vi "Create Type.vi"(6 "Searchable Attributes":string[](array[string]), 8 "error in (no error)":errorcluster, 9 "Description":string, 10 "Name":string, 11 "IoT Session in":refnum<class "IoT Session.lvclass">) -> (0 "error out":errorcluster, 3 "IoT Session out":refnum<class "IoT Session.lvclass">)   [LabVIEW 2015, in "NI_AWS_IoT.lvlib" / "IoT Session.lvclass"]
uses:
  IoT Session.lvclass
  Core/HTTP Request/Valid String Specification.ctl
  Core/HTTP Request/Request Options.ctl
  Core/HTTP Request/Name Value Pair.ctl
  Core/HTTP Request/Region handling.ctl
  Core/HTTP Request/URL formatting.ctl
  Core/HTTP Request/HTTP Request.lvclass
  JSON Parsing/NI_JSON Parsing.lvlib
panel:
  out "Created Type ARN":string
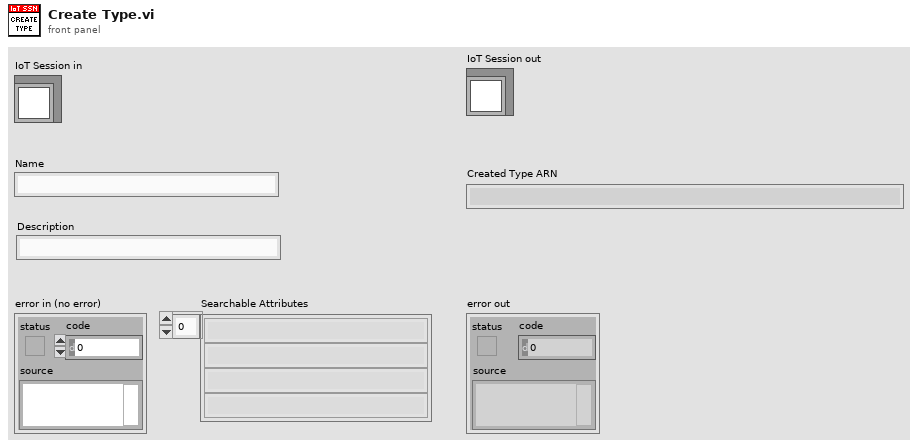
[diagram p1: front panel]
types:
  T1 = typedef "NI_AWS_Core.lvlib/HTTP Request.lvclass/Valid String Specification.ctl" = enum16{"none", "only [alphanumeric][-][_]", "only [alphanumeric][-][_][space]", "phone number +1xxxyyyzzzz", "Regular Expression"}
  T2 = typedef "NI_AWS_Core.lvlib/HTTP Request.lvclass/Name Value Pair.ctl" = cluster{"name":string, "value":string}
  T3 = typedef "NI_AWS_Core.lvlib/HTTP Request.lvclass/Request Options.ctl" = cluster{"request headers":T2[], "request parameters":T2[], "request body":string, "region handling":T4, "URL formatting":T5}
  T4 = typedef "NI_AWS_Core.lvlib/HTTP Request.lvclass/Region handling.ctl" = enum16{"use region everywhere", "use region (authentication only)", "use region (URL only)", "ignore region everwhere"}
  T5 = typedef "NI_AWS_Core.lvlib/HTTP Request.lvclass/URL formatting.ctl" = enum16{"region-", "region."}
  T6 = typedef "NI_AWS_Core.lvlib/HTTP Request.lvclass/Response.ctl" = cluster{"Headers":string, "Body":string}
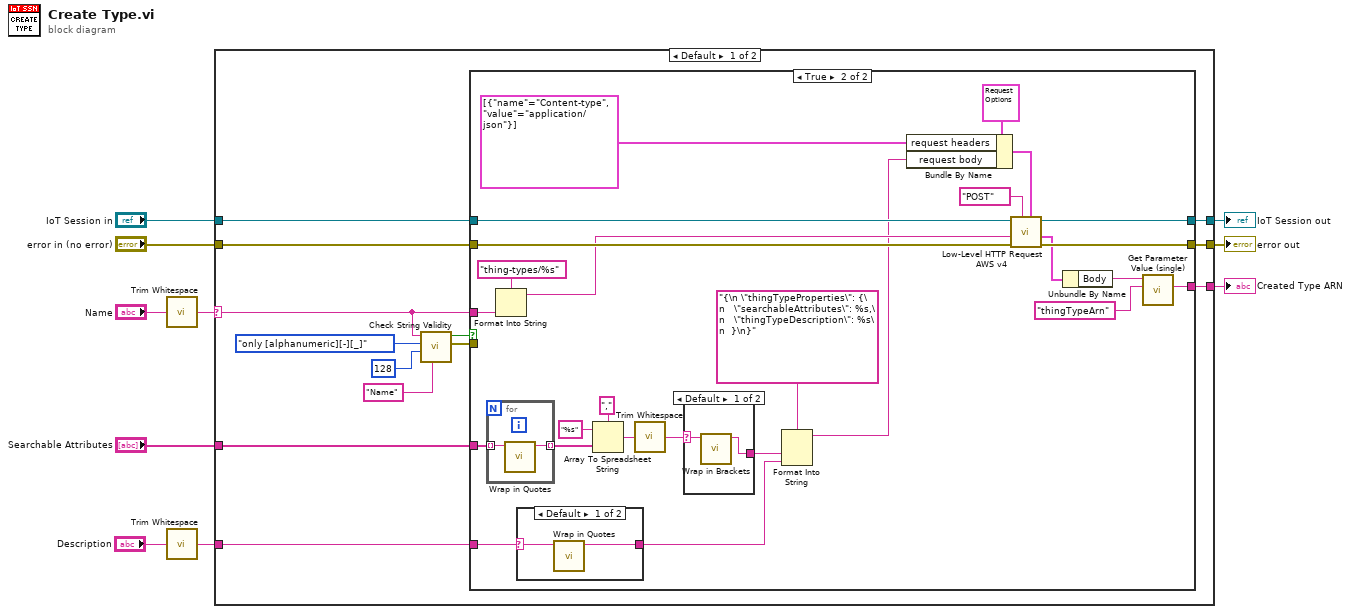
[diagram p0: block diagram]
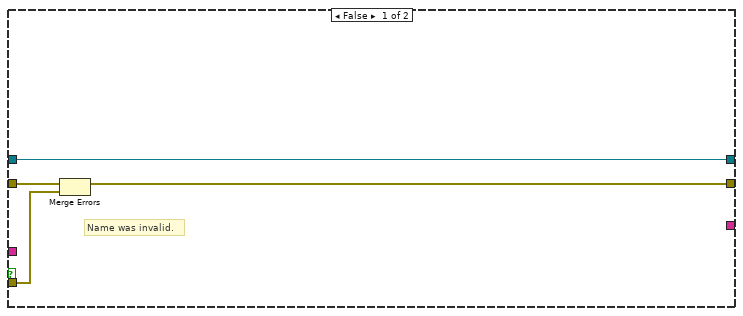
[diagram p2: hidden frame]
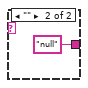
[diagram p3: hidden frame]
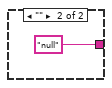
[diagram p4: hidden frame]
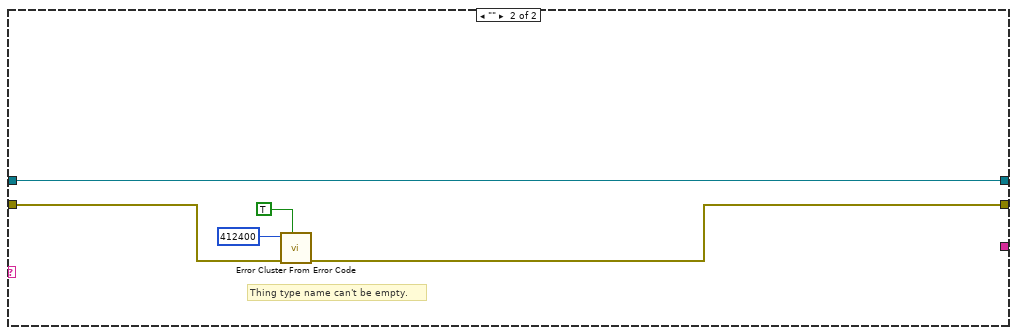
[diagram p5: hidden frame]
diagram:
  n1 = call <vilib>:"Trim Whitespace.vi"("string"="Name") -> ("trimmed string"=w6:string)  [unwired: 1 in]
  n2 = call <vilib>:"Trim Whitespace.vi"("string"="Description") -> ("trimmed string"=w5:string)  [unwired: 1 in]
  n3 = case shown="Default" w6 {
    selector: w6 -> [w16 _]
    tunnel: "error in (no error)" -> [w23 w66]
    tunnel: [w22 w65] -> w9
    tunnel: [w21 w63] -> w8
    tunnel: w5 -> [w12 _]
    tunnel: "IoT Session in" -> [w14 w63]
    tunnel: "Searchable Attributes" -> [w13 _]
    tunnel: [w11 _] -> w1
    frame Default {
      n4 = call "Check String Validity.vi"("String Name for Error"="Name", "Max Characters"=128, "Valid String Specification"=Valid_String_Specification."only [alphanumeric][-][_]", "String"=w16) -> ("string error"=w17:errorcluster, "Valid"=w15:bool)  [unwired: 6 in]
      n5 = case shown="True" w15 {
        tunnel: w23 -> [w27 w53]
        tunnel: [w26 w52] -> w22
        tunnel: [w24 w51] -> w21
        tunnel: w16 -> [_ w47]
        tunnel: w17 -> [w25 _]
        tunnel: w14 -> [w24 w43]
        tunnel: w12 -> [_ w40]
        tunnel: w13 -> [_ w38]
        tunnel: [_ w28] -> w11
        frame False {
          # "Name was invalid."
          n6 = Merge Errors(w27, w25) -> (w26:errorcluster)
        }
        frame True {
          n7 = for {
            tunnel: w38 -> [w58] mode=indexing
            tunnel: [w57] -> w37 mode=indexing
            n8 = call "Wrap in Quotes.vi"("String"=w58) -> ("String with Quotes"=w57:string)  [unwired: 10 in]
          }
          n9 = Format Into String(format string="thing-types/%s", w47) -> (resulting string=w48:string)  [unwired: 2 in, 1 out]
          n10 = case shown="Default" w40 {
            selector: w40 -> [w60 _]
            tunnel: [w59 "null"] -> w39
            frame Default {
              n11 = call "Wrap in Quotes.vi"("String"=w60) -> ("String with Quotes"=w59:string)  [unwired: 10 in]
            }
            frame "" {
            }
          }
          n12 = Array To Spreadsheet String(delimiter (Tab)=",", array=w37, 3:"%s") -> (spreadsheet string=w34:string)
          n13 = call <vilib>:"Trim Whitespace.vi"("string"=w34) -> ("trimmed string"=w33:string)  [unwired: 1 in]
          n14 = case shown="Default" w33 {
            selector: w33 -> [w55 _]
            tunnel: [w54 "null"] -> w32
            frame Default {
              n15 = call "Wrap in Brackets.vi"("String"=w55) -> ("String with Brackets"=w54:string)  [unwired: 10 in]
            }
            frame "" {
            }
          }
          n16 = Format Into String(format string="{\n \"thingTypeProperties\": {\n   \"searchableAttributes\": %s,\n   \"thingTypeDescription\": %s\n  }\n}", w32, w39) -> (resulting string=w41:string)  [unwired: 2 in, 1 out]
          n17 = Bundle By Name(cluster=T3 {"request headers"=[], "request parameters"=[], "request body"="", "region handling"=enum."use region everywhere", "URL formatting"=enum."region."} ("Request Options"), "request headers"=T2[] [{"name"="Content-type", "value"="application/json"}], "request body"=w41) -> (w45:T3)
          n18 = call "Low-Level HTTP Request AWS v4.vi"("Request Options"=w45, "HTTP-Verb"="POST", "error in (no error)"=w53, "URL Suffix"=w48, "AWS Core in"=w43) -> ("error out"=w52:errorcluster, "Response"=w31:T6, "AWS Core out"=w51:refnum<class "IoT Session.lvclass">)  [unwired: 3 in, 1 out]
          n19 = Unbundle By Name(w31) -> ("Body"=w30:string)
          n20 = call "Get Parameter Value (single).vi"("Parameter Name"="thingTypeArn", "JSON"=w30) -> ("Parameter Value"=w28:string)  [unwired: 6 in, 3 out]
        }
      }
    }
    frame "" {
      # "Thing type name can't be empty."
      n21 = call <vilib>:"Error Cluster From Error Code.vi"("show call chain? (False)"=TRUE, "error in (no error)"=w66, "error code (0)"=412400) -> ("error out"=w65:errorcluster)  [unwired: 6 in]
    }
  }
  "error out" <- w9
  "IoT Session out" <- w8
  "Created Type ARN" <- w1
